vi "Position Listbox.vi"(8 "error in (no error)":errorcluster, 10 "Listbox placement":T1, 11 "Refs":T2) -> (0 "error out":errorcluster)   [LabVIEW 2021, in "Autocomplete Textbox.lvlib"]
uses:
  Autocomplete Textbox.lvlib
  Refs.ctl
  Classes/Handle/Listbox placement.ctl
  Classes/Handle/Handle.lvclass
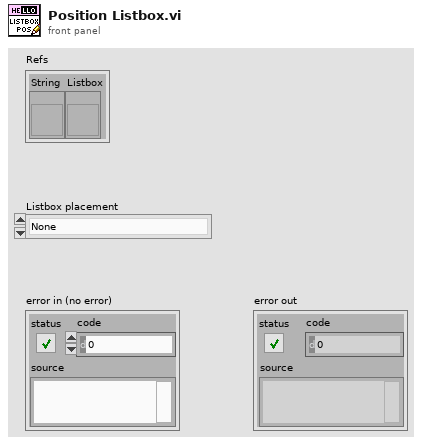
[diagram p1: front panel]
types:
  T1 = typedef "Autocomplete Textbox.lvlib/Handle.lvclass/Listbox placement.ctl" = enum16{"None", "Under String", "Fit to Pane"}
  T2 = typedef "Autocomplete Textbox.lvlib/Refs.ctl" = cluster{"String":refnum<vi>, "Listbox":refnum<vi>}
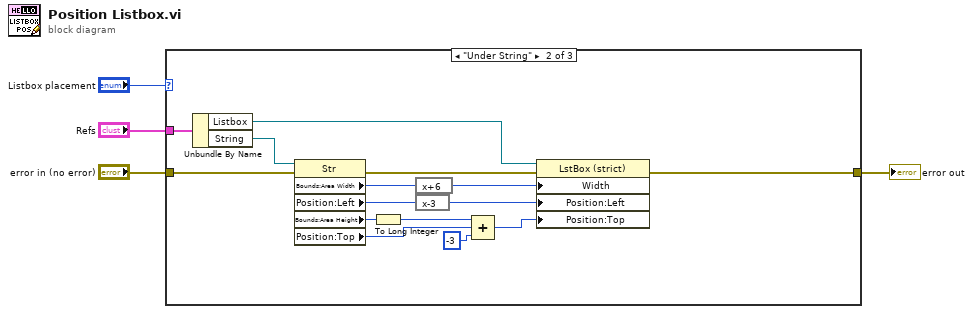
[diagram p0: block diagram]
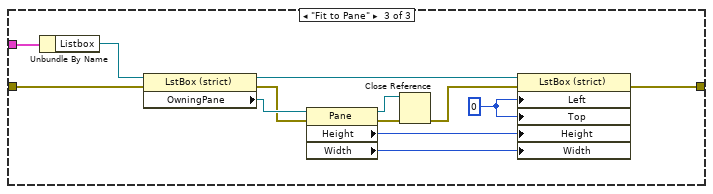
[diagram p3: hidden frame]
diagram:
  n1 = case shown="\"Under String\"" "Listbox placement" {
    tunnel: "error in (no error)" -> [w5 w11 w27]
    tunnel: [w5 w9 w21] -> w3
    tunnel: "Refs" -> [_ w8 w33]
    frame "None" {
    }
    frame "Under String" {
      n2 = Unbundle By Name(w8) -> ("Listbox"=w6:refnum<vi>, "String"=w7:refnum<vi>)
      n3 = property on="Property Node" class="Str"(reference=w7, error in=w11) -> (error out=w10:errorcluster, "Bounds:Area Width"=w13:u32, "Position:Left"=w15:i32, "Bounds:Area Height"=w20:u32, "Position:Top"=w19:i32)  [unwired: 1 out]
      n4 = To Long Integer(number=w20) -> (32bit integer=w16:i32)
      n5 = expression code="x+6"(w13) -> (w12:u32)
      n6 = expression code="x-3"(w15) -> (w14:i32)
      n7 = Compound Arithmetic op=ADD(w16, w19, -3 ("value")) -> (w18:i32)
      n8 = property on="Property Node" class="LstBox (strict)"(reference=w6, error in=w10, "Width"=w12, "Position:Left"=w14, "Position:Top"=w18) -> (error out=w9:errorcluster)  [unwired: 1 out]
    }
    frame "Fit to Pane" {
      w30 = 0 ("Position:Left")
      n9 = Unbundle By Name(w33) -> ("Listbox"=w22:refnum<vi>)
      n10 = property class="LstBox (strict)"(reference=w22, error in=w27) -> (reference out=w31:refnum<vi>, error out=w26:errorcluster, "OwningPane"=w32:refnum<vi>)
      n11 = property class="Pane"(reference=w32, error in=w26) -> (reference out=w25:refnum<vi>, error out=w24:errorcluster, "Height"=w29:u32, "Width"=w28:u32)
      n12 = Close Reference(reference=w25, error in (no error)=w24) -> (error out=w23:errorcluster)
      n13 = property class="LstBox (strict)"(reference=w31, error in=w23, "Left"=w30, "Top"=w30, "Height"=w29, "Width"=w28) -> (error out=w21:errorcluster)  [unwired: 1 out]
    }
  }
  "error out" <- w3
